vi "Send Update Active Wheel Command.vi"(8 "error in (no error)":errorcluster, 10 "active wheel index":i32, 11 "subpanel to main command event":T1) -> (0 "error out":errorcluster)   [LabVIEW 2017, in "NI_Robotics_Configure Steering Frame.lvlib"]
uses:
  <vilib>/robotics/Dialog/Configure Steering Frame/NI_Robotics_Configure Steering Frame.lvlib
  <vilib>/robotics/Dialog/Configure Steering Frame/Subpanel to Main Command Event.ctl
  <vilib>/robotics/Dialog/Configure Steering Frame/Subpanel to Main Command.ctl
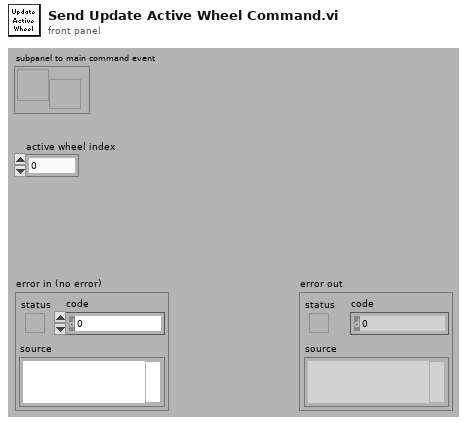
[diagram p1: front panel]
types:
  T1 = typedef "NI_Robotics_Configure Steering Frame.lvlib/Subpanel to Main Command Event.ctl" = refnum<user-event>
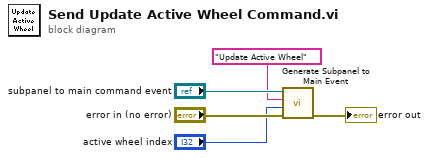
[diagram p0: block diagram]
diagram:
  n1 = call <vilib>:"Generate Subpanel to Main Event.vi"("error in (no error)"="error in (no error)", "data"="active wheel index", "command"="Update Active Wheel", "subpanel to main command event"="subpanel to main command event") -> ("error out"=→"error out":errorcluster)  [unwired: 7 in]
